vi "server.Format LV Error as JSON Data.vi"(10 "error in":errorcluster) -> (0 "error out":errorcluster, 2 "Error Value out":refnum<class "JSON Value.lvclass">)   [LabVIEW 2016, in "JSONRPC Server.lvclass"]
doc: "This converts a LabVIEW Error to a JSON Tree for use with \"Add Response - Server Error\"."
uses:
  JSONRPC Server.lvclass
  <vilib>/NI/JSON Support for LabVIEW/JSON Value/JSON Value.lvclass
  <vilib>/NI/JSON Support for LabVIEW/JSON Value/New JSON Value/New JSON ({}).vi
  <vilib>/NI/JSON Support for LabVIEW/JSON Value/Object/Insert Value/Insert Value (Numeric).vi
  <vilib>/NI/JSON Support for LabVIEW/JSON Value/Object/Insert Value/Insert Value (String).vi
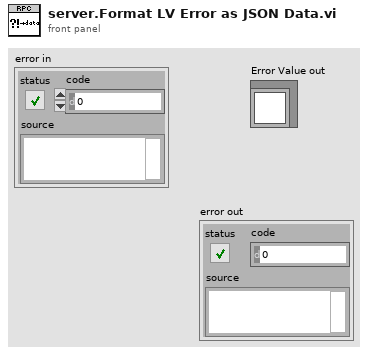
[diagram p1: front panel]
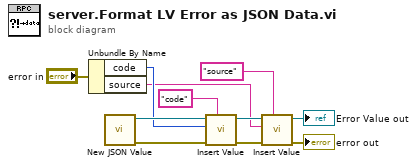
[diagram p0: block diagram]
diagram:
  n1 = Unbundle By Name("error in") -> ("code"=w4:i32, "source"=w2:string)
  n2 = call-poly <vilib>:"New JSON Value.vi"() -> ("error out"=w5:errorcluster, "JSON Value out"=w10:refnum<class "JSON Value.lvclass">)  [unwired: 10 in]
  n3 = call-poly <vilib>:"Insert Value.vi"("key"="code" ("Name"), "error in (no error)"=w5, "value"=w4, "JSON Value in"=w10) -> ("error out"=w6:errorcluster, "JSON Value out"=w9:refnum<class "JSON Value.lvclass">)  [unwired: 5 in, 1 out]
  n4 = call-poly <vilib>:"Insert Value.vi"("key"="source" ("Name"), "error in (no error)"=w6, "value"=w2, "JSON Value in"=w9) -> ("error out"=→"error out":errorcluster, "JSON Value out"=→"Error Value out":refnum<class "JSON Value.lvclass">)  [unwired: 5 in, 1 out]
